vi "DEV SN To DAQmx Device Name.vi"(8 "error in (no error)":errorcluster, 11 "USN_DEV (JSON)":string) -> (0 "error out":errorcluster, 3 "DAQmx Device Name":tag)   [LabVIEW 2015]
uses:
  Share Data/uPower_kit.ctl
  <resource>/objmgr/daqmx.rc
panel:
  out "DevNames":tag[](array[tag])
  out "DevSerialNum":u32
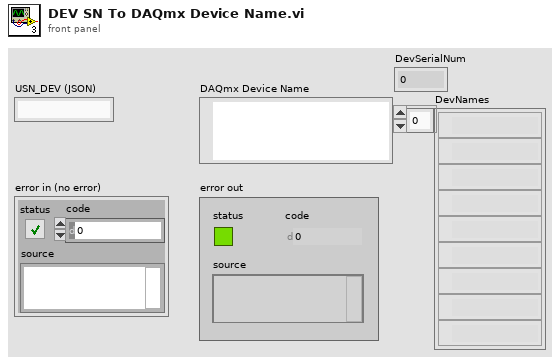
[diagram p1: front panel]
types:
  T1 = typedef "uPower_kit.ctl" = cluster{"DEV":string, "BUSY":bool, "VBAT":dbl, "OUTPUT":bool, "LAST_RESULT":dbl, "DURATION":u16, "TRIGGER":bool, "RANGE":string, "Vsource":dbl, "FW":string, "Mode":string}
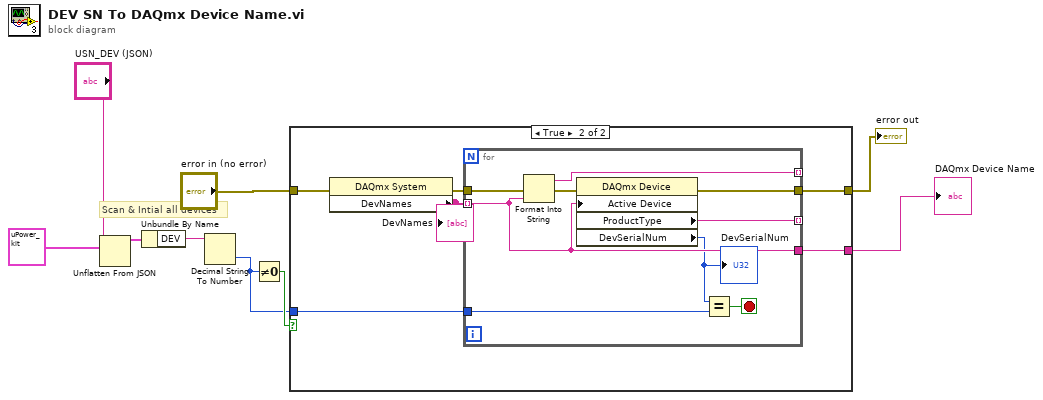
[diagram p0: block diagram]
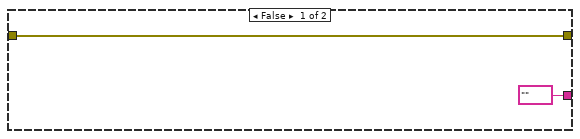
[diagram p2: hidden frame]
diagram:
  # "Scan & Intial all devices"
  n1 = Unflatten From JSON(JSON string="USN_DEV (JSON)", type and defaults=T1 {"DEV"="", "BUSY"=FALSE, "VBAT"=0.0, "OUTPUT"=FALSE, "LAST_RESULT"=0.0, "DURATION"=0, "TRIGGER"=FALSE, "RANGE"="", "Vsource"=0.0, "FW"="", "Mode"=""} ("DEV_BUSY")) -> (value=w1:T1)  [unwired: 5 in, 1 out]
  n2 = Unbundle By Name(w1) -> ("DEV"=w6:string)
  n3 = Decimal String To Number(string=w6) -> (number=w8:i32)  [unwired: 2 in, 1 out]
  n4 = Not Equal To 0?(x=w8) -> (x != 0?=w9:bool)
  n5 = case shown="True" w9 {
    tunnel: "error in (no error)" -> [w11 w17]
    tunnel: [w11 w16] -> w4
    tunnel: [tag "" w13] -> w5
    tunnel: w8 -> [_ w12]
    frame False {
    }
    frame True {
      n6 = property class="DAQmx System"(error in=w17) -> (error out=w15:errorcluster, "DevNames"=w14:tag[])  [unwired: 1 in, 1 out]
      "DevNames" <- w14
      n7 = for {
        tunnel: w14 -> [w24] mode=indexing
        tunnel: [w26] -> _ mode=indexing
        tunnel: [w25] -> _ mode=indexing
        tunnel: [w24] -> w13
        tunnel: w15 -> [w22]
        tunnel: [w21] -> w16
        tunnel: w12 -> [w19]
        stop <- w18 stop-if-true
        n8 = Format Into String(error in=w22, w24) -> (resulting string=w25:string, error out=w23:errorcluster)  [unwired: 2 in]
        n9 = property class="DAQmx Device"(error in=w23, "Active Device"=w24) -> (error out=w21:errorcluster, "ProductType"=w26:string, "DevSerialNum"=w20:u32)  [unwired: 1 in, 1 out]
        "DevSerialNum" <- w20
        n10 = Equal?(x=w20, y=w19) -> (x = y?=w18:bool)
      }
    }
  }
  "error out" <- w4
  "DAQmx Device Name" <- w5
